vi "Percent Drive.vi"(8 "error in (no error)":errorcluster, 10 "Y Joystick":dbl, 11 "X Joystick":dbl) -> (0 "error out":errorcluster)   [LabVIEW 2017, in "Drive Train.lvlib"]
uses:
  Drive Train.lvlib
  <vilib>/Rock Robotics/WPI/ThirdParty/Phoenix-LabVIEW/Motor Controller/Controls/CTRE_Phoenix_MotorControl_ControlMode.ctl
  Controls/FGV Actions.ctl
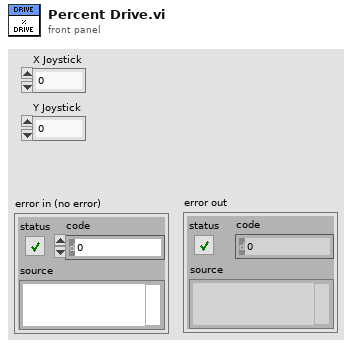
[diagram p1: front panel]
types:
  T1 = typedef "Drive Train.lvlib/FGV Actions.ctl" = enum16{"Get", "Set"}
  T2 = typedef "CTRE_Phoenix_MotorControl_ControlMode.ctl" = u16
  T3 = typedef "Drive Train.lvlib/Library Information.ctl" = cluster{"Right Motor Name":string, "Left Motor Name":string, "Current Control Mode":T2, "Motion Magic Parameters":T4, "Motor Controllers Parameters":T5}
  T4 = typedef "Drive Train.lvlib/Motion Magic Parameters.ctl" = cluster{"Native Units":dbl}
  T5 = typedef "Drive Train.lvlib/Motor Controllers Parameters.ctl" = cluster{"Max Current (amps)":i32, "PID Buckets":cluster{"High Gear":i32, "High Gear Ramp":i32, "Low Gear":i32, "Low Gear Ramp":i32}}
  T6 = typedef "WPI_MotorControlDeviceRef.ctl" = cluster{"DeviceStatus":errorcluster, "Type":T7, "PWM":cluster{"PWM Channel":T8, "DeadBand":T9}, "CAN":cluster{"Device Number":u8, "SetOutput VI Ref":variant, "GetOutput VI Ref":variant, "Enable VI Ref":variant, "Disable VI Ref":variant, "Data":variant}, "Invert":bool, "DIO PWM":cluster{"PWM \"Enable\" Channel":T8, "DIOChannel":T10, "PWM Rate":dbl}}
  T7 = typedef "WPI_MotorControlType.ctl" = enum16{"PWM", "CAN", "DIO PWM"}
  T8 = typedef "FPGA_DIOPWMChannel.ctl" = enum8{"PWM 0", "PWM 1", "PWM 2", "PWM 3", "PWM 4", "PWM 5", "PWM 6", "PWM 7", "PWM 8", "PWM 9", "PWM MXP 0", "PWM MXP 1", "PWM MXP 2", "PWM MXP 3", "PWM MXP 4", "PWM MXP 5", "PWM MXP 6", "PWM MXP 7", "PWM MXP 8", "PWM MXP 9", "Invalid"}
  T9 = typedef "WPI_PWMDeadband.ctl" = cluster{"Name":string, "maxPositivePwm":i32, "minPositivePwm":i32, "centerPwm":i32, "maxNegativePwm":i32, "minNegativePwm":i32, "angularRange":u16}
  T10 = typedef "FPGA_DIOChannel.ctl" = enum8{"DIO 0", "DIO 1", "DIO 2", "DIO 3", "DIO 4", "DIO 5", "DIO 6", "DIO 7", "DIO 8", "DIO 9", "DIO MXP 0", "DIO MXP 1", "DIO MXP 2", "DIO MXP 3", "DIO MXP 4", "DIO MXP 5", "DIO MXP 6", "DIO MXP 7", "DIO MXP 8", "DIO MXP 9", "DIO MXP 10", "DIO MXP 11", "DIO MXP 12", "DIO MXP 13", "DIO MXP 14", "DIO MXP 15", "SPI Port CS1", "SPI Port CS2", "SPI Port CS3", "SPI Port MISO", "SPI Port MOSI", "Invalid"}
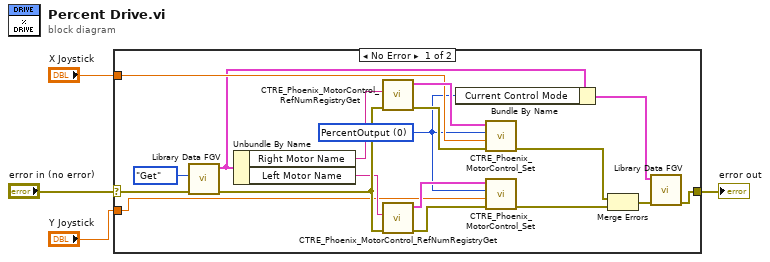
[diagram p0: block diagram]
diagram:
  n1 = case shown="No Error" "error in (no error)" {
    selector: "error in (no error)" -> [w13 w23]
    tunnel: [w8 w23] -> w3
    tunnel: "X Joystick" -> [w11 _]
    tunnel: "Y Joystick" -> [w10 _]
    frame No Error {
      w5 = T2 0 items=["PercentOutput"=0, "Position"=1, "Velocity"=2, "Current"=3, "Follower"=5, "MotionProfile"=6, "MotionMagic"=7, "MotionMagicArc"=8, "MotionProfileArc"=10, "Disabled"=15] ("Control Mode")
      n2 = call "Library Data FGV.vi"("error in (no error)"=w13, "FGV Actions"=FGV_Actions."Get") -> ("error out"=w21:errorcluster, "Library Information out"=w7:T3)  [unwired: 8 in]
      n3 = Unbundle By Name(w7) -> ("Right Motor Name"=w16:string, "Left Motor Name"=w17:string)
      n4 = call <vilib>:"CTRE_Phoenix_MotorControl_RefNumRegistryGet.vi"("error in (no error)"=w21, "refnum name"=w16) -> ("error out"=w19:errorcluster, "PhoenixMotorControlDevRef"=w20:T6)  [unwired: 8 in]
      n5 = call <vilib>:"CTRE_Phoenix_MotorControl_RefNumRegistryGet.vi"("error in (no error)"=w21, "refnum name"=w17) -> ("error out"=w22:errorcluster, "PhoenixMotorControlDevRef"=w18:T6)  [unwired: 8 in]
      n6 = Bundle By Name(cluster=w7, "Current Control Mode"=w5) -> (w6:T3)
      n7 = call <vilib>:"CTRE_Phoenix_MotorControl_Set.vi"("error in (no error)"=w19, "Output"=w11, "Control Mode"=w5, "PhoenixMotorControlDevRef"=w20) -> ("error out"=w14:errorcluster)  [unwired: 6 in, 1 out]
      n8 = call <vilib>:"CTRE_Phoenix_MotorControl_Set.vi"("error in (no error)"=w22, "Output"=w10, "Control Mode"=w5, "PhoenixMotorControlDevRef"=w18) -> ("error out"=w15:errorcluster)  [unwired: 6 in, 1 out]
      n9 = Merge Errors(w14, w15) -> (w9:errorcluster)
      n10 = call "Library Data FGV.vi"("error in (no error)"=w9, "Library Information in"=w6) -> ("error out"=w8:errorcluster)  [unwired: 8 in, 1 out]
    }
    frame Error {
    }
  }
  "error out" <- w3
